vi "IncrCurveInd.vi"(8 "error in (no error)":errorcluster caption="entrée d'erreur (pas d'erreur)", 11 "Interface en entrée":refnum<class "Interface.lvclass"> caption="DNL_LabVIEW Object in") -> (0 "error out":errorcluster caption="sortie d'erreur", 3 "Interface en sortie":refnum<class "Interface.lvclass"> caption="DNL_LabVIEW Object out")   [LabVIEW 2019, in "Interface.lvclass"]
uses:
  Interface.lvclass
  Interface.lvclass/Interface.ctl
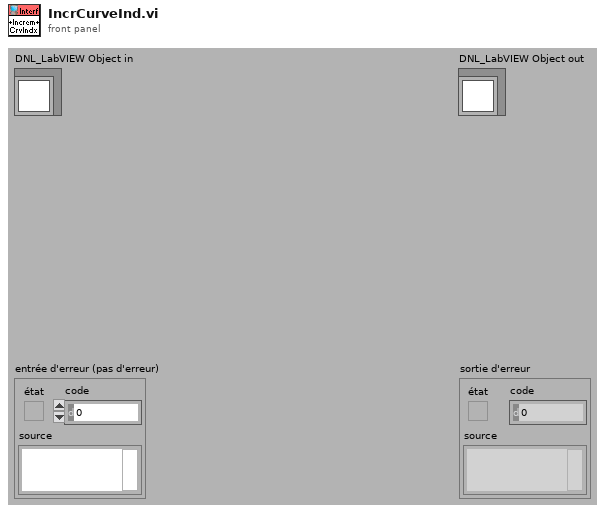
[diagram p1: front panel]
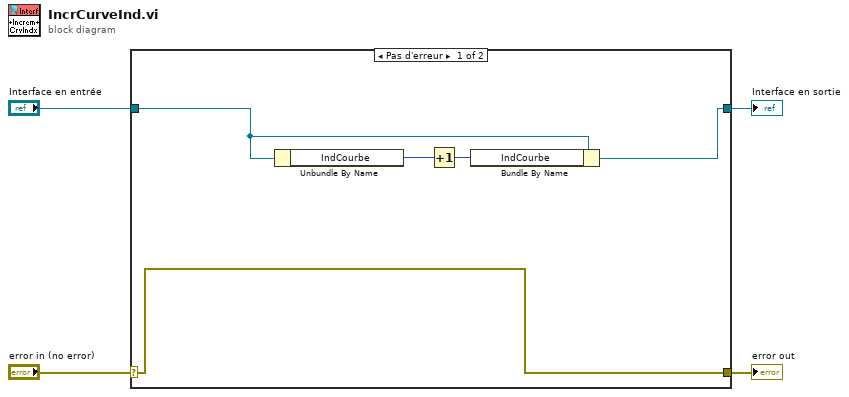
[diagram p0: block diagram]
diagram:
  n1 = case shown="Pas d'erreur" "error in (no error)" {
    selector: "error in (no error)" -> [w5 w11]
    tunnel: [w5 w11] -> w3
    tunnel: [w6 w10] -> w1
    tunnel: "Interface en entrée" -> [w7 w10]
    frame No Error {
      n2 = Unbundle By Name(w7) -> ("IndCourbe"=w9:i64)
      n3 = Increment(x=w9) -> (x+1=w8:i64)
      n4 = Bundle By Name(cluster=w7, "IndCourbe"=w8) -> (w6:refnum<class "Interface.lvclass">)
    }
    frame Error {
    }
  }
  "error out" <- w3
  "Interface en sortie" <- w1
